vi "Initialize.vi"(8 "error in (no error)":errorcluster, 11 "device data model in":refnum<class "WebSocket Data Model.lvclass">) -> (0 "error out":errorcluster, 3 "device data model out":refnum<class "WebSocket Data Model.lvclass">)   [LabVIEW 2021, in "WebSockets.lvlib" / "WebSocket Data Model.lvclass"]
doc: "This VI initializes the device data model."
uses:
  WebSocket Data Model.lvclass
  Type Definitions/Data Model.ctl
  WebSocket Data Model.lvclass/WebSocket Data Model.ctl
  Modbus_v121c/Data Model/Device Data Model.lvclass
  WebSocket/Opcodes.ctl
  WebSocket/WebSocket.lvclass
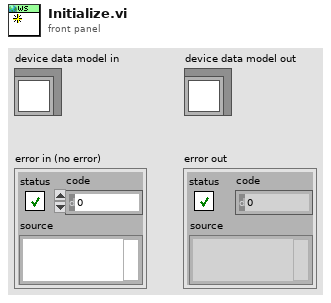
[diagram p1: front panel]
types:
  T1 = typedef "WebSockets.lvlib/WebSocket Data Model.lvclass/Data Model.ctl" = cluster{"UTC":u64, "Receive Binary Data":u8[], "Receive Text Data":string, "Send Binary Data":u8[], "Send Text Data":string, "ES":u8}
  T2 = typedef "WebSockets.lvlib/WebSocket.lvclass/Opcodes.ctl" = u8
  T3 = typedef "Device Data Model.lvclass/N channel.ctl" = cluster{"N DI channel":i32, "N DO channel":i32, "N AI channel":i32, "N AO channel":i32}
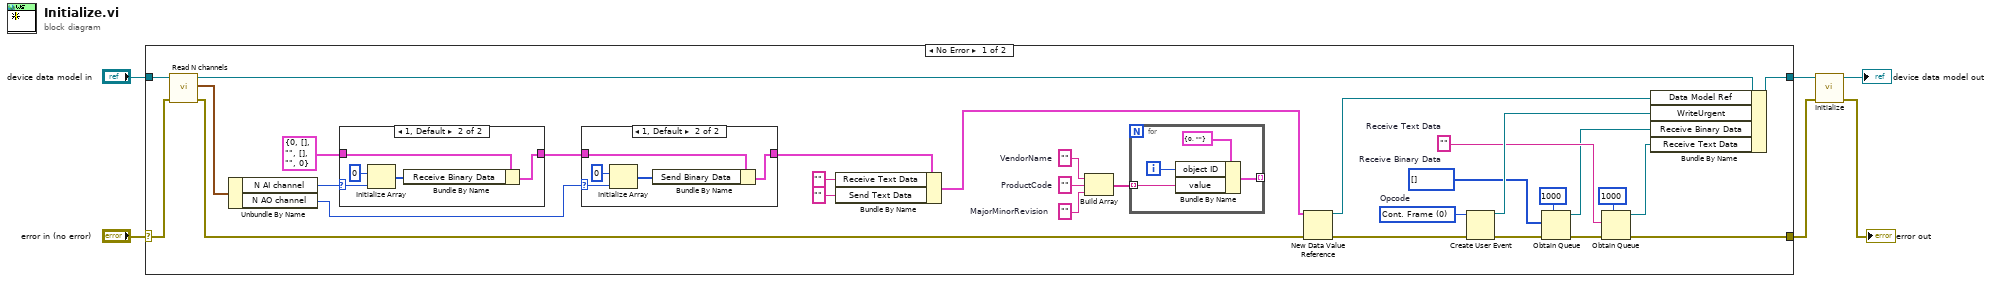
[diagram p0: block diagram]
diagram:
  n1 = case shown="No Error" "error in (no error)" {
    selector: "error in (no error)" -> [w29 w54]
    tunnel: "device data model in" -> [w30 w55]
    tunnel: [w12 w54] -> w5
    tunnel: [w33 w55] -> w4
    frame No Error {
      w11 = ""  # Receive Text Data
      w10 = u8[] []  # Receive Binary Data
      w15 = T2 0 items=["Cont. Frame", "Text", "Binary", "Close Frame", "Ping", "Pong"]  # Opcode
      w35 = ""  # MajorMinorRevision
      w37 = ""  # ProductCode
      w36 = ""  # VendorName
      n2 = call-dynamic "Read N channels.vi"("error in (no error)"=w29, "device data model in"=w30) -> ("error out"=w28:errorcluster, "N channel"=w18:T3, "device data model out"=w31:refnum<class "WebSocket Data Model.lvclass">)  [unwired: 7 in]
      n3 = Unbundle By Name(w18) -> ("N AI channel"=w26:i32, "N AO channel"=w17:i32)
      n4 = case shown="1, Default" w26 {
        selector: w26 -> [_ w45]
        tunnel: T1 {"UTC"=0, "Receive Binary Data"=[], "Receive Text Data"="", "Send Binary Data"=[], "Send Text Data"="", "ES"=0} ("Data Model") -> [w44 w48]
        tunnel: [w44 w46] -> w20
        frame 0 {
        }
        frame 1, Default {
          n5 = Initialize Array(u8 0 ("Boolean"), w45) -> (w47:u8[])
          n6 = Bundle By Name(cluster=w48, "Receive Binary Data"=w47) -> (w46:T1)
        }
      }
      n7 = case shown="1, Default" w17 {
        selector: w17 -> [_ w39]
        tunnel: w20 -> [w38 w42]
        tunnel: [w38 w40] -> w19
        frame 0 {
        }
        frame 1, Default {
          n8 = Initialize Array(u8 0 ("Boolean"), w39) -> (w41:u8[])
          n9 = Bundle By Name(cluster=w42, "Send Binary Data"=w41) -> (w40:T1)
        }
      }
      n10 = Bundle By Name(cluster=w19, "Receive Text Data"="" ("Text Data"), "Send Text Data"="" ("Text Data")) -> (w25:T1)
      n11 = Build Array(w36, w37, w35) -> (w34:string[])
      n12 = for {
        tunnel: w34 -> [w51] mode=indexing
        tunnel: [w50] -> _ mode=indexing
        i -> [w52]
        n13 = Bundle By Name(cluster=cluster{"object ID":u8, "value":string} {"object ID"=0, "value"=""} ("Cluster"), "object ID"=w52, "value"=w51) -> (w50:cluster{"object ID":u8, "value":string})
      }
      n14 = New Data Value Reference(data value=w25, error in=w28) -> (data value reference=w32:refnum<data-value>, error out=w23:errorcluster)
      n15 = Create User Event(user event datatype=w15, error in=w23) -> (user event=w22:refnum<user-event>, error out=w16:errorcluster)
      n16 = Obtain Queue(max queue size (-1, unlimited)=1000, element data type=w10, error in (no error)=w16) -> (queue out=w8:refnum<queue>, error out=w13:errorcluster)  [unwired: 2 in, 1 out]
      n17 = Obtain Queue(max queue size (-1, unlimited)=1000, element data type=w11, error in (no error)=w13) -> (queue out=w7:refnum<queue>, error out=w12:errorcluster)  [unwired: 2 in, 1 out]
      n18 = Bundle By Name(cluster=w31, "Data Model Ref"=w32, "WriteUrgent"=w22, "Receive Binary Data"=w8, "Receive Text Data"=w7) -> (w33:refnum<class "WebSocket Data Model.lvclass">)
    }
    frame Error {
    }
  }
  n19 = call-parent "Initialize.vi"("error in"=w5, "device data model in"=w4) -> ("error out"=→"error out":errorcluster, "device data model out"=→"device data model out":refnum<class "WebSocket Data Model.lvclass">)  [unwired: 8 in]
